vi "G#BaseAggregator_Create.vi"(0 "reference in":refnum<class "G#BaseAggregator.lvclass">, 3 "control values":variant[](array[variant]), 5 "error in (no error)":errorcluster) -> (14 "reference out":refnum<class "G#BaseAggregator.lvclass">, 19 "error out":errorcluster)   [LabVIEW 2010, in "G#BaseAggregator.lvclass"]
doc: "Constructor."
uses:
  G#BaseAggregator.lvclass
  G#SubSubClass1_class/G#SubSubClass1.lvclass
  <vilib>/addons/_AddQ/G#Object/G#Object.lvclass
  G#SubSubClass2_class/G#SubSubClass2.lvclass
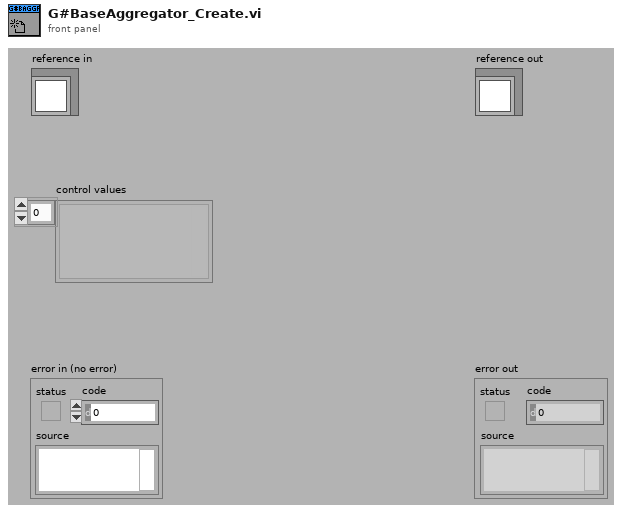
[diagram p1: front panel]
types:
  T1 = typedef "G#BaseAggregator.lvclass/ObjectAttributesRef.ctl" = refnum<data-value>
  T2 = typedef "G#BaseAggregator.lvclass/ObjectAttributes.ctl" = cluster{"Numeric":dbl, "G#BaseClass1.lvclass":refnum<class "G#BaseClass1.lvclass">, "G#BaseClass2.lvclass":refnum<class "G#BaseClass2.lvclass">}
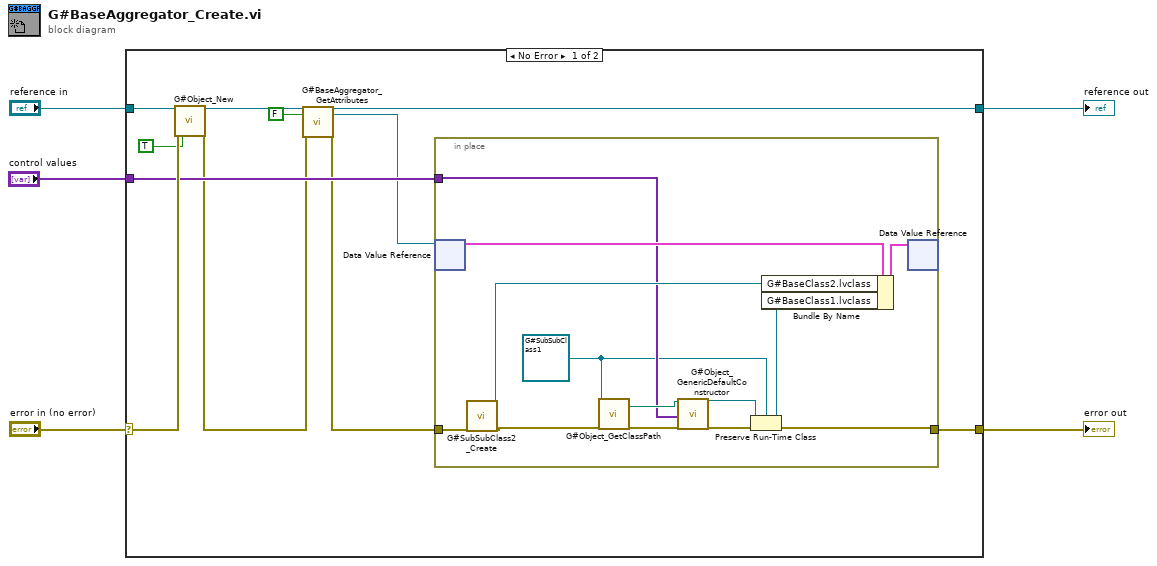
[diagram p0: block diagram]
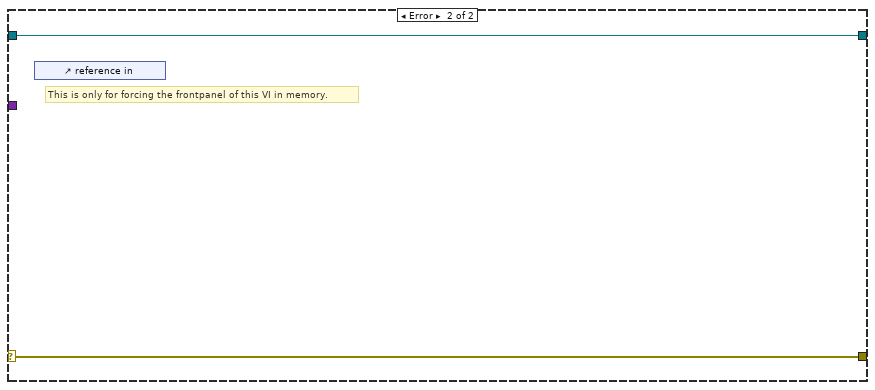
[diagram p2: hidden frame]
diagram:
  n1 = case shown="No Error" "error in (no error)" {
    selector: "error in (no error)" -> [w15 w31]
    tunnel: [w13 w31] -> w4
    tunnel: [w10 w30] -> w2
    tunnel: "reference in" -> [w16 w30]
    tunnel: "control values" -> [w12 _]
    frame No Error {
      n2 = call <vilib>:"G#Object_New.vi"("reference in"=w16, "error in (no error)"=w15, "user counter (T)?"=TRUE ("User Counter")) -> ("reference out"=w11:refnum<class "G#BaseAggregator.lvclass">, "error out"=w9:errorcluster)  [unwired: 14 in, 1 out]
      n3 = call "G#BaseAggregator_GetAttributes.vi"("reference in"=w11, "return data? (T)"=FALSE, "error in (no error)"=w9) -> ("reference out"=w10:refnum<class "G#BaseAggregator.lvclass">, "attributes ref"=w7:T1, "error out"=w8:errorcluster)  [unwired: 13 in, 1 out]
      n4 = in-place {
        in-place-border: w8 -> [w27]
        in-place-border: [w20] -> w13
        in-place-border: w12 -> [w22]
        w18 = refnum<class "G#SubSubClass1.lvclass"> refnum ("G#SubSubClass1.lvclass")
        n5 = in-place-dvr #1(w7) -> (w29:T2)  [unwired: 1 out]
        n6 = call "G#SubSubClass2_Create.vi"("error in (no error)"=w27) -> ("reference out"=w26:refnum<class "G#SubSubClass2.lvclass">, "error out"=w25:errorcluster)  [unwired: 17 in]
        n7 = call-dynamic "G#Object_GetClassPath.vi"("reference in"=w18, "error in (no error)"=w25) -> ("class path"=w23:path, "error out"=w24:errorcluster)  [unwired: 15 in, 1 out]
        n8 = call <vilib>:"G#Object_GenericDefaultConstructor.vi"("class path"=w23, "control values"=w22, "error in (no error)"=w24) -> ("reference out"=w19:refnum<class "G#Object.lvclass">, "error out"=w21:errorcluster)  [unwired: 14 in, 1 out]
        n9 = Preserve Run-Time Class(object in=w19, error in=w21, 2:w18) -> (object out=w17:refnum<class "G#SubSubClass1.lvclass">, error out=w20:errorcluster)
        n10 = Bundle By Name(cluster=w29, "G#BaseClass2.lvclass"=w26, "G#BaseClass1.lvclass"=w17) -> (w28:T2)
        n11 = in-place-dvr #1(w28) -> ()  [unwired: 2 out]
      }
    }
    frame Error {
      # "This is only for forcing the frontpanel of this VI in memory."
      n12 = control-ref of="reference in"() -> ()  [unwired: 1 out]
    }
  }
  "error out" <- w4
  "reference out" <- w2
